vi "MSG New Data For Display.vi"(8 "error in":errorcluster, 10 "Payload":variant) -> (0 "error out":errorcluster)   [LabVIEW 2020, in "GUI.lvlib"]
uses:
  GUI.lvlib
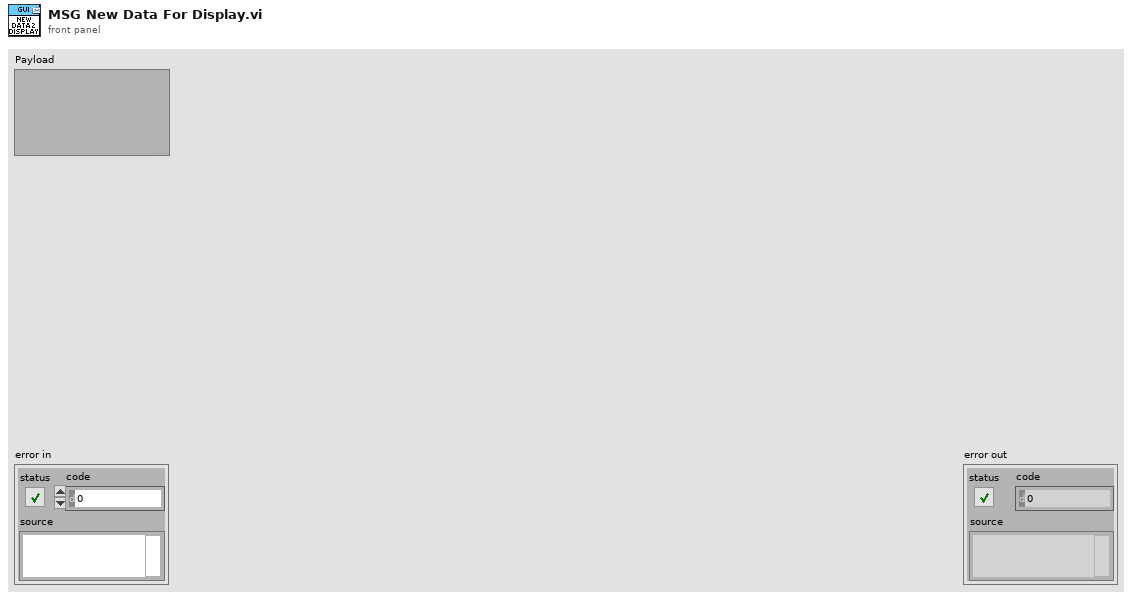
[diagram p1: front panel]
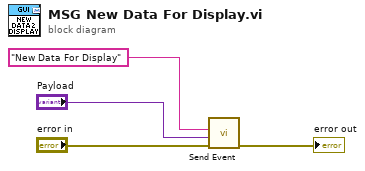
[diagram p0: block diagram]
diagram:
  n1 = call "Send Event.vi"("error in"="error in", "Payload"="Payload", "Command"="New Data For Display") -> ("error out"=→"error out":errorcluster)  [unwired: 8 in]
